vi "Assign Value.vi"(8 "error in (no error)":errorcluster, 10 "Assigned Value":refnum<class "Abs_Value.lvclass">, 11 "Abs_Extended Float in":refnum<class "Abs_Extended Float.lvclass">) -> (0 "error out":errorcluster, 3 "Abs_Extended Float out":refnum<class "Abs_Extended Float.lvclass">)   [LabVIEW 2021, in "Abs_Extended Float.lvclass"]
uses:
  Abs_Extended Float.lvclass
  Value/Abs_Value.lvclass
  Numeric/Abs_Numeric.lvclass
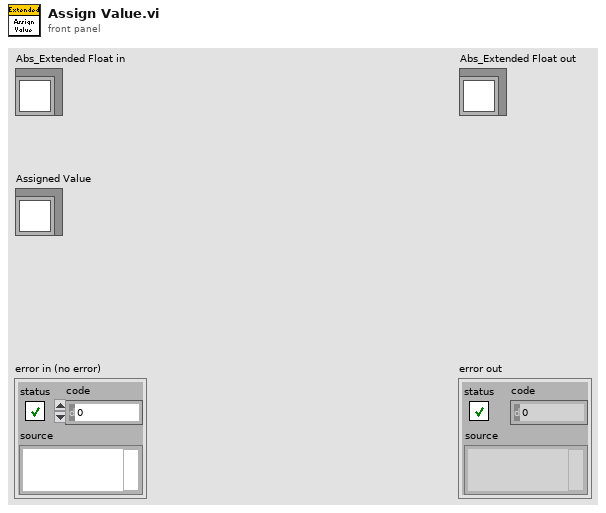
[diagram p1: front panel]
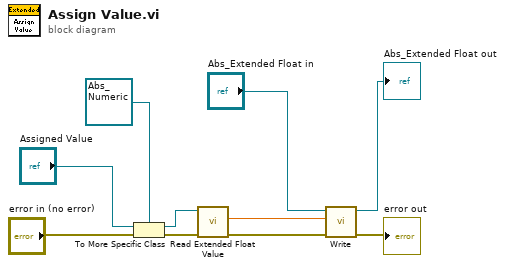
[diagram p0: block diagram]
diagram:
  n1 = To More Specific Class(target class=refnum<class "Abs_Numeric.lvclass"> refnum ("Abs_Numeric.lvclass"), reference="Assigned Value", error in="error in (no error)") -> (specific class reference=w7:refnum<class "Abs_Numeric.lvclass">, error out=w6:errorcluster)
  n2 = call-dynamic "Read Extended Float Value.vi"("error in (no error)"=w6, "Numeric in"=w7) -> ("error out"=w5:errorcluster, "Extended Float"=w4:ext)  [unwired: 7 in, 1 out]
  n3 = call-dynamic "Write.vi"("error in (no error)"=w5, "Value"=w4, "Double Float.lvclass_340760 in"="Abs_Extended Float in") -> ("error out"=→"error out":errorcluster, "Double Float.lvclass_340760 out"=→"Abs_Extended Float out":refnum<class "Abs_Extended Float.lvclass">)  [unwired: 7 in]
